vi "FTW-Test-Router-Shutdown.vi"() -> (0 "Test Result":errorcluster)   [LabVIEW 2014]
uses:
  src/core/actor/router/FTW-Router.lvclass
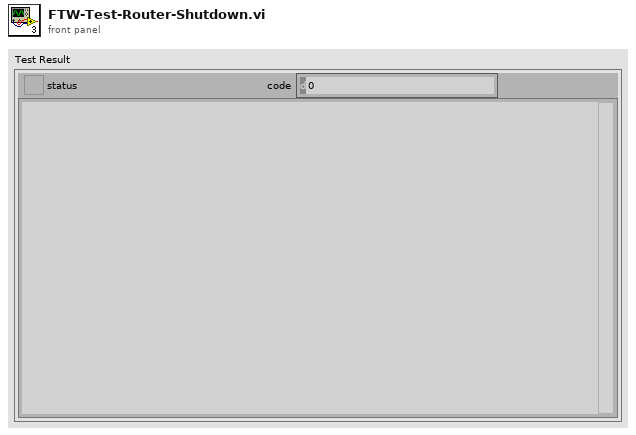
[diagram p1: front panel]
types:
  T1 = cluster{"[0]":refnum<event-registration>, "[1]":refnum<event-registration>, "[2]":refnum<event-registration>, "[3]":refnum<event-registration>, "[4]":refnum<event-registration>, "[5]":refnum<event-registration>, "[6]":refnum<event-registration>, "[7]":refnum<event-registration>, "[8]":refnum<event-registration>, "[9]":refnum<event-registration>, "[10]":refnum<event-registration>, "[11]":refnum<event-registration>, "[12]":refnum<event-registration>, "[13]":refnum<event-registration>, "[14]":refnum<event-registration>, "[15]":refnum<event-registration>, "[16]":refnum<event-registration>, "[17]":refnum<event-registration>, "[18]":refnum<event-registration>, "[19]":refnum<event-registration>, "[20]":refnum<event-registration>, "[21]":refnum<event-registration>, "[22]":refnum<event-registration>, "[23]":refnum<event-registration>, "[24]":refnum<event-registration>, "[25]":refnum<event-registration>, "[26]":refnum<event-registration>, "[27]":refnum<event-registration>, "[28]":refnum<event-registration>, "[29]":refnum<event-registration>, "[30]":refnum<event-registration>, "[31]":refnum<event-registration>}
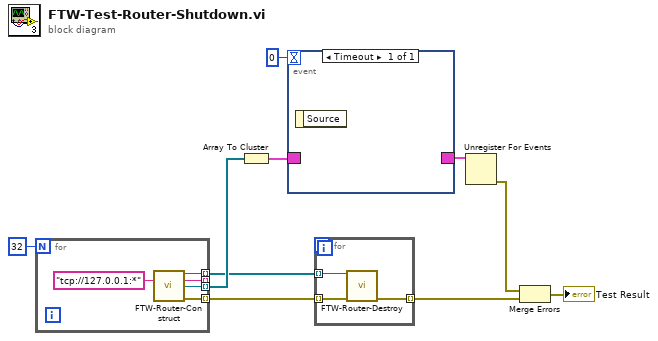
[diagram p0: block diagram]
diagram:
  n1 = for {
    N: 32 -> [_]
    tunnel: [w14] -> w6 mode=indexing
    tunnel: [w13] -> _ mode=indexing
    tunnel: [w12] -> w9 mode=indexing
    tunnel: [w11] -> w5 mode=indexing
    n2 = call "FTW-Router-Construct.vi"("Inbox Address"="tcp://127.0.0.1:*") -> ("FTW Router"=w14:refnum<class "FTW-Router.lvclass">, "Resolved Inbox Address"=w13:string, "Incoming Message"=w12:refnum<event-registration>, "error out"=w11:errorcluster)  [unwired: 11 in]
  }
  n3 = Array To Cluster(array=w9) -> (cluster=w8:T1)
  n4 = event shown="[0] Timeout" {
    selector: w8 -> [_]
    dyn-events: [_] -> w7
    timeout: 0 -> [_]
    event Timeout {
      n5 = event-data() -> ()  [unwired: 1 in, 1 out]
    }
  }
  n6 = for {
    tunnel: w6 -> [w18] mode=indexing
    tunnel: w5 -> [w17] mode=indexing
    tunnel: [w16] -> w4 mode=indexing
    n7 = call "FTW-Router-Destroy.vi"("FTW Router"=w18, "error in"=w17) -> ("error out"=w16:errorcluster)  [unwired: 13 in]
  }
  n8 = Unregister For Events(event registration refnum=w7) -> (error out=w1:errorcluster)  [unwired: 1 in]
  n9 = Merge Errors(w1, w4) -> (→"Test Result":errorcluster)
